vi "Check polymorh script.vi"(8 "Multipl factor":i32=9, 9 "Limits":T2={"min synth f"=9.0, "max synth f"=14.0, "Ramp limits [mT/s]"=[7.5, 5.0, 3.5, 2.5, 1.5], "Field ranges [T]"=[3.0, 9.6, 13.3, 15.0, 16.0]}, 10 "New val":T1={"Start"=0.0, "Start Caption"="Start [T]", "End"=0.0, "End Caption"="End [T]", "Sweep"=0.0, "Sweep caption"="Rate [mT/s]", "Constant"=0.0, "Constant caption"="Freq [GHz]", "Mod_F [kHz]"=0.1, "Mod_A [G]"=0.0, "Tau [ms]"=0.0, "Positioners [mm|°]"=[], "Tmp [K]"=0.0, "Wait [min]"=0.0, "Carousel"=-1, "Comment"="", "Auto-mod"=TRUE, "Execute"=FALSE} {"Carousel" items=["0", "1", "2", "3", "4", "5", "6"]; "Positioners [mm|°]" min=-1.0 max=330.0; "Tau [ms]" min=0.002 max=10000.0; "Wait [min]" min=0.0 max=3000.0; "Tmp [K]" min=0.0 max=350.0; "Mod_A [G]" min=0.0 max=100.0; "Mod_F [kHz]" min=0.1 max=150.0}, 11 "Old val":T1={"Start"=0.0, "Start Caption"="Start [T]", "End"=0.0, "End Caption"="End [T]", "Sweep"=0.0, "Sweep caption"="Rate [mT/s]", "Constant"=0.0, "Constant caption"="Freq [GHz]", "Mod_F [kHz]"=0.1, "Mod_A [G]"=0.0, "Tau [ms]"=0.0, "Positioners [mm|°]"=[], "Tmp [K]"=0.0, "Wait [min]"=0.0, "Carousel"=-1, "Comment"="", "Auto-mod"=TRUE, "Execute"=FALSE} {"Carousel" items=["0", "1", "2", "3", "4", "5", "6"]; "Positioners [mm|°]" min=-1.0 max=330.0; "Tau [ms]" min=0.002 max=10000.0; "Wait [min]" min=0.0 max=3000.0; "Tmp [K]" min=0.0 max=350.0; "Mod_A [G]" min=0.0 max=100.0; "Mod_F [kHz]" min=0.1 max=150.0}) -> (3 "Row out":T1={"Start"=0.0, "Start Caption"="Start [T]", "End"=0.0, "End Caption"="End [T]", "Sweep"=0.0, "Sweep caption"="Rate [mT/s]", "Constant"=0.0, "Constant caption"="Freq [GHz]", "Mod_F [kHz]"=0.1, "Mod_A [G]"=0.0, "Tau [ms]"=0.0, "Positioners [mm|°]"=[], "Tmp [K]"=0.0, "Wait [min]"=0.0, "Carousel"=-1, "Comment"="", "Auto-mod"=TRUE, "Execute"=FALSE} {"Carousel" items=["0", "1", "2", "3", "4", "5", "6"]; "Positioners [mm|°]" min=-1.0 max=330.0; "Tau [ms]" min=0.002 max=10000.0; "Wait [min]" min=0.0 max=3000.0; "Tmp [K]" min=0.0 max=350.0; "Mod_A [G]" min=0.0 max=100.0; "Mod_F [kHz]" min=0.1 max=150.0})   [LabVIEW 2022 SP3]
uses:
  Datatypes/script polymorh line.ctl
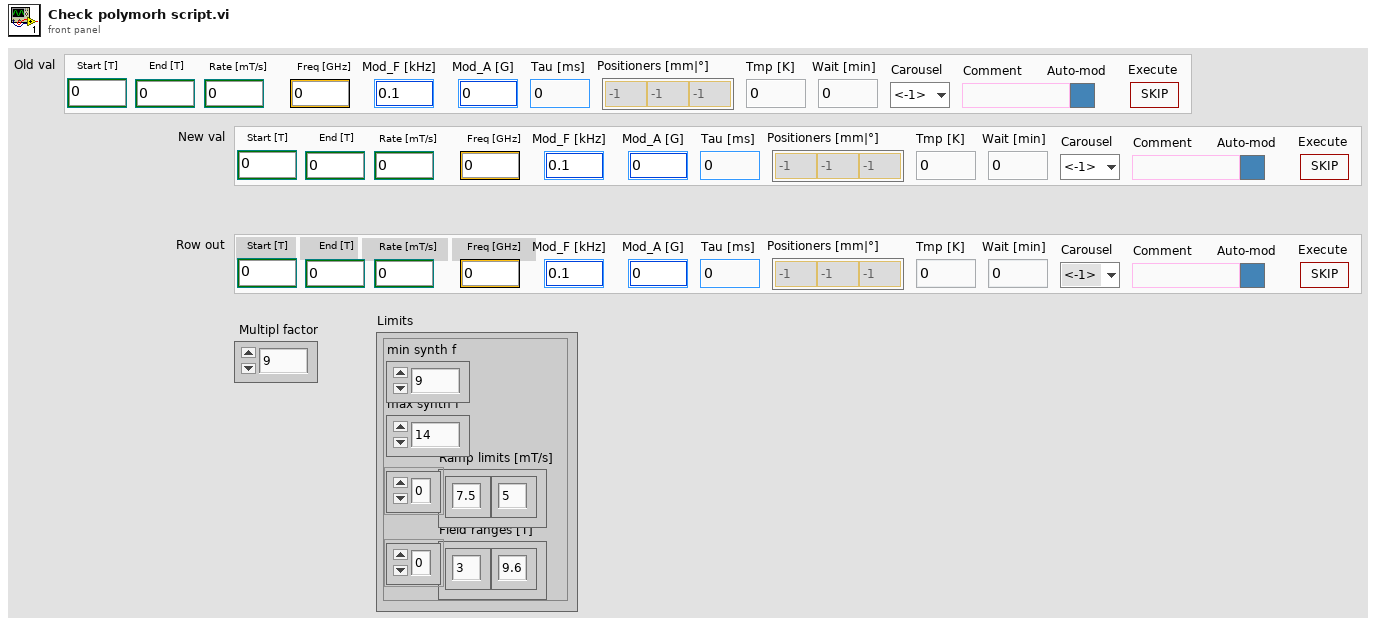
[diagram p1: front panel]
types:
  T1 = typedef "script polymorh line.ctl" = cluster{"Start":dbl, "Start Caption":string, "End":dbl, "End Caption":string, "Sweep":dbl, "Sweep caption":string, "Constant":dbl, "Constant caption":string, "Mod_F [kHz]":dbl, "Mod_A [G]":dbl, "Tau [ms]":dbl, "Positioners [mm|°]":dbl[], "Tmp [K]":dbl, "Wait [min]":dbl, "Carousel":i8, "Comment":string, "Auto-mod":bool, "Execute":bool}
  T2 = cluster{"min synth f":dbl, "max synth f":dbl, "Ramp limits [mT/s]":dbl[], "Field ranges [T]":dbl[]}
  T3 = cluster{"Start":bool, "Start Caption":bool, "End":bool, "End Caption":bool, "Sweep":bool, "Sweep caption":bool, "Constant":bool, "Constant caption":bool, "Mod_F [kHz]":bool, "Mod_A [G]":bool, "Tau [ms]":bool, "Positioners [mm|°]":bool[], "Tmp [K]":bool, "Wait [min]":bool, "Carousel":bool, "Comment":bool, "Auto-mod":bool, "Execute":bool}
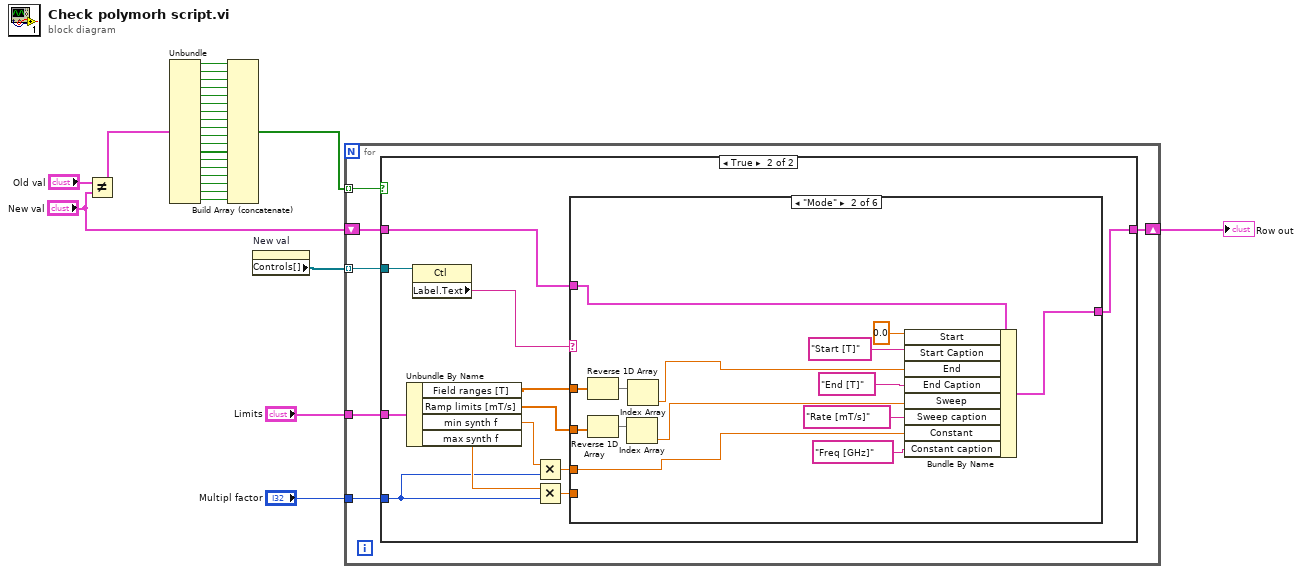
[diagram p0: block diagram]
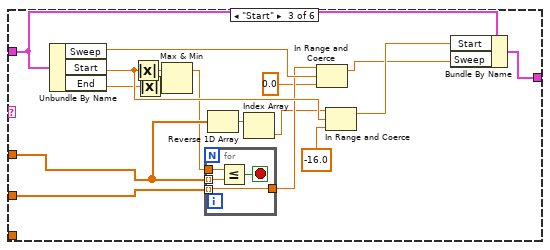
[diagram p4: hidden frame]
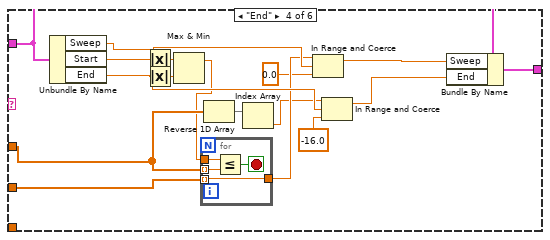
[diagram p5: hidden frame]
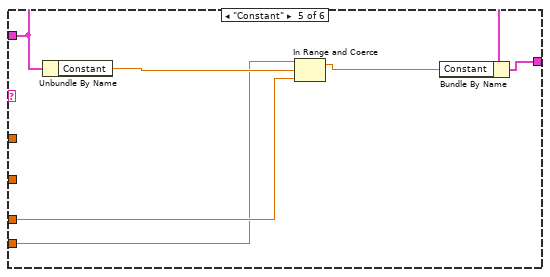
[diagram p6: hidden frame]
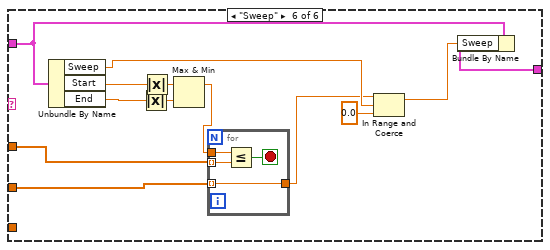
[diagram p7: hidden frame]
diagram:
  n1 = Not Equal?(x="Old val", y="New val") -> (x != y?=w19:T3)
  n2 = Unbundle(w19) -> ("Start"=w18:bool, "Start Caption"=w17:bool, "End"=w16:bool, "End Caption"=w15:bool, "Sweep"=w14:bool, "Sweep caption"=w7:bool, "Constant"=w8:bool, "Constant caption"=w9:bool, "Mod_F [kHz]"=w10:bool, "Mod_A [G]"=w11:bool, "Tau [ms]"=w12:bool, "Positioners [mm|°]"=w13:bool[], "Tmp [K]"=w6:bool, "Wait [min]"=w5:bool, "Carousel"=w4:bool, "Comment"=w3:bool, "Auto-mod"=w2:bool, "Execute"=w1:bool)
  n3 = Build Array (concatenate)(w18, w17, w16, w15, w14, w7, w8, w9, w10, w11, w12, w13, w6, w5, w4, w3, w2, w1) -> (w24:bool[])
  n4 = property on="New val" class="Clust (strict)"() -> ("Controls[]"=w20:refnum<vi>[])  [unwired: 2 in, 2 out]
  n5 = for {
    tunnel: w20 -> [w32] mode=indexing
    tunnel: w24 -> [w31] mode=indexing
    shift-right: [w29] -> w21
    shift-left: "New val" -> [w30]
    tunnel: "Multipl factor" -> [w28]
    tunnel: "Limits" -> [w27]
    n6 = case shown="True" w31 {
      tunnel: w32 -> [_ w45]
      tunnel: w30 -> [w33 w43]
      tunnel: [w33 w42] -> w29
      tunnel: w28 -> [_ w35]
      tunnel: w27 -> [_ w34]
      frame False {
      }
      frame True {
        n7 = Unbundle By Name(w34) -> ("Field ranges [T]"=w40:dbl[], "Ramp limits [mT/s]"=w41:dbl[], "min synth f"=w38:dbl, "max synth f"=w39:dbl)
        n8 = property class="Ctl"(reference=w45) -> ("Label.Text"=w44:string)  [unwired: 1 in, 2 out]
        n9 = Multiply(x=w38, y=w35) -> (x*y=w37:dbl)
        n10 = Multiply(x=w39, y=w35) -> (x*y=w36:dbl)
        n11 = case shown="\"Mode\"" w44 {
          tunnel: w43 -> [w46 w60 w76 w97 w108 w121]
          tunnel: [w46 w59 w74 w95 w107 w120] -> w42
          tunnel: w40 -> [_ w58 w73 w91 _ w117]
          tunnel: w41 -> [_ w55 w72 w94 _ w116]
          tunnel: w37 -> [_ w52 _ _ w104 _]
          tunnel: w36 -> [_ _ _ _ w103 _]
          frame "Ignore", Default {
          }
          frame "Mode" {
            n12 = Reverse 1D Array(array=w58) -> (reversed array=w57:dbl[])
            n13 = Reverse 1D Array(array=w55) -> (reversed array=w56:dbl[])
            n14 = Index Array(array=w56) -> (element=w53:dbl)  [unwired: 1 in]
            n15 = Index Array(array=w57) -> (element=w54:dbl)  [unwired: 1 in]
            n16 = Bundle By Name(cluster=w60, "Start"=0.0 ("Rate[GHz/s]"), "Start Caption"="Start [T]", "End"=w54, "End Caption"="End [T]", "Sweep"=w53, "Sweep caption"="Rate [mT/s]", "Constant"=w52, "Constant caption"="Freq [GHz]") -> (w59:T1)
          }
          frame "Start" {
            n17 = Unbundle By Name(w76) -> ("Sweep"=w77:dbl, "Start"=w70:dbl, "End"=w69:dbl)
            n18 = Absolute Value(x=w70) -> (abs(x)=w63:dbl)
            n19 = Absolute Value(x=w69) -> (abs(x)=w62:dbl)
            n20 = Max & Min(x=w63, y=w62) -> (max(x,y)=w68:dbl)  [unwired: 1 out]
            n21 = for {
              tunnel: w68 -> [w81]
              tunnel: w73 -> [w80] mode=indexing
              tunnel: w72 -> [w79] mode=indexing
              tunnel: [w79] -> w67
              stop <- w78 stop-if-true
              n22 = Less Or Equal?(x=w81, y=w80) -> (x <= y?=w78:bool)
            }
            n23 = Reverse 1D Array(array=w73) -> (reversed array=w66:dbl[])
            n24 = Index Array(array=w66) -> (element=w65:dbl)  [unwired: 1 in]
            n25 = In Range and Coerce(upper limit=w67, x=w77, lower limit=0.0) -> (coerced(x)=w71:dbl)  [unwired: 1 out]
            n26 = In Range and Coerce(upper limit=w65, x=w70, lower limit=-16.0) -> (coerced(x)=w75:dbl)  [unwired: 1 out]
            n27 = Bundle By Name(cluster=w76, "Start"=w75, "Sweep"=w71) -> (w74:T1)
          }
          frame "End" {
            n28 = Unbundle By Name(w97) -> ("Sweep"=w98:dbl, "Start"=w92:dbl, "End"=w93:dbl)
            n29 = Absolute Value(x=w92) -> (abs(x)=w83:dbl)
            n30 = Absolute Value(x=w93) -> (abs(x)=w84:dbl)
            n31 = Max & Min(x=w83, y=w84) -> (max(x,y)=w89:dbl)  [unwired: 1 out]
            n32 = for {
              tunnel: w89 -> [w102]
              tunnel: w91 -> [w101] mode=indexing
              tunnel: w94 -> [w100] mode=indexing
              tunnel: [w100] -> w88
              stop <- w99 stop-if-true
              n33 = Less Or Equal?(x=w102, y=w101) -> (x <= y?=w99:bool)
            }
            n34 = Reverse 1D Array(array=w91) -> (reversed array=w86:dbl[])
            n35 = Index Array(array=w86) -> (element=w85:dbl)  [unwired: 1 in]
            n36 = In Range and Coerce(upper limit=w88, x=w98, lower limit=0.0) -> (coerced(x)=w96:dbl)  [unwired: 1 out]
            n37 = In Range and Coerce(upper limit=w85, x=w93, lower limit=-16.0) -> (coerced(x)=w90:dbl)  [unwired: 1 out]
            n38 = Bundle By Name(cluster=w97, "Sweep"=w96, "End"=w90) -> (w95:T1)
          }
          frame "Constant" {
            n39 = Unbundle By Name(w108) -> ("Constant"=w106:dbl)
            n40 = In Range and Coerce(upper limit=w103, x=w106, lower limit=w104) -> (coerced(x)=w105:dbl)  [unwired: 1 out]
            n41 = Bundle By Name(cluster=w108, "Constant"=w105) -> (w107:T1)
          }
          frame "Sweep" {
            n42 = Unbundle By Name(w121) -> ("Sweep"=w114:dbl, "Start"=w119:dbl, "End"=w118:dbl)
            n43 = Absolute Value(x=w118) -> (abs(x)=w109:dbl)
            n44 = Absolute Value(x=w119) -> (abs(x)=w110:dbl)
            n45 = Max & Min(x=w110, y=w109) -> (max(x,y)=w113:dbl)  [unwired: 1 out]
            n46 = for {
              tunnel: w113 -> [w125]
              tunnel: w117 -> [w124] mode=indexing
              tunnel: w116 -> [w123] mode=indexing
              tunnel: [w123] -> w112
              stop <- w122 stop-if-true
              n47 = Less Or Equal?(x=w125, y=w124) -> (x <= y?=w122:bool)
            }
            n48 = In Range and Coerce(upper limit=w112, x=w114, lower limit=0.0) -> (coerced(x)=w115:dbl)  [unwired: 1 out]
            n49 = Bundle By Name(cluster=w121, "Sweep"=w115) -> (w120:T1)
          }
        }
      }
    }
  }
  "Row out" <- w21
